vi "Create Array of Points.vi"(0 "rx output divider":T1, 5 "horizontal step size":i16=1, 7 "vertical step size":i16=1, 11 "error in":errorcluster) -> (4 "array of points":T2[][](array[typedef]), 15 "error out":errorcluster)   [LabVIEW 2014, in "niHighSpeedSerial Rectangular Eye Scan Point Iterator v1 Host.lvclass"]
doc: "Creates the array of points to measure based on the passed in parameters.\n\n<B>Input Parameters</B>\n\n<B>rx output divider</B> represents the configuration of the receiver output divider. This should match the values configured with RXRATE and RXOUT_DIV.\nenum values: 1,2,4,8,16\n\n<B>horizontal step size</B> is the number of offsets to skip between each point on the horizontal axis.\n\n<B>vertical step size</B> is the number of offsets to skip between each point on the vertical axis.\n\n<B>error in</B> describes error conditions that occur before this node runs. This input provides standard 'error in' functionality.\n\n<B>Output Parameters</B>\n\n<B>array of points</B> contains information related to each point, including its offsets, bit error rate, sample count, and error rate.\n\n<B>array of points.point offsets</B> contains the horizontal and vertical offsets for a point.\n\n<B>array of points.point offsets.horizontal offset</B> is the horizontal (unit interval) offset of a point.\n\n<B>array of points.point offsets.vertical offset</B> is the vertical (uncalibrated voltage) offset of a point.\n\n<B>array of points.sample count</B> is the number of samples measured.\n\n<B>array of points.error count</B> is the number of errors detected while measuring the point.\n\n<B>array of points.bit error rate</B> is the calculated statistical bit error rate based on the number of error counts and sample counts received.\n\n<B>error out</B> contains error information. This output provides standard 'error out' functionality."
uses:
  <instrlib>/niHighSpeedSerial/Eye Scan/v1/Host/Impl/Rect Iter/niHighSpeedSerial Rectangular Eye Scan Point Iterator v1 Host.lvclass
  <instrlib>/niHighSpeedSerial/Eye Scan/v1/Host/Common/Public/Point.ctl
  <instrlib>/niHighSpeedSerial/Eye Scan/v1/Host/Common/Public/Point Offsets.ctl
  <instrlib>/niHighSpeedSerial/Eye Scan/v1/Host/Common/Public/RX Output Divider.ctl
  <instrlib>/niHighSpeedSerial/Eye Scan/v1/Host/Common/niHighSpeedSerial Eye Scan Common v1 Host.lvlib
panel:
  out "size(s)":i32[](array[numeric])
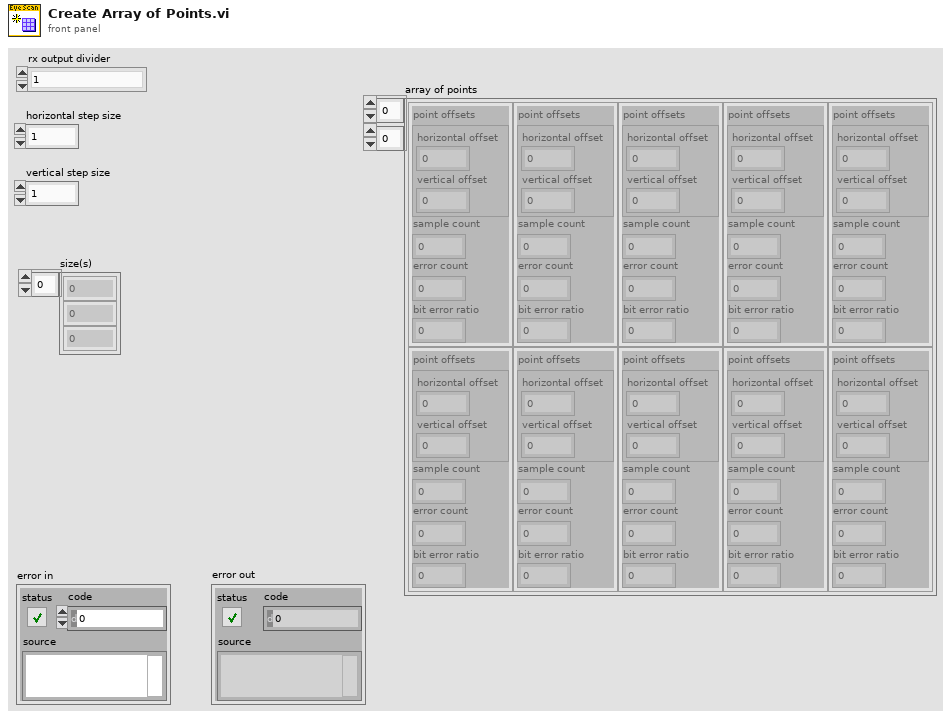
[diagram p1: front panel]
types:
  T1 = typedef "niHighSpeedSerial Eye Scan Common v1 Host.lvlib/RX Output Divider.ctl" = enum16{"1", "2", "4", "8", "16"}
  T2 = typedef "niHighSpeedSerial Eye Scan Common v1 Host.lvlib/Point.ctl" = cluster{"point offsets":T3, "sample count":u64, "error count":u64, "bit error ratio":dbl}
  T3 = typedef "niHighSpeedSerial Eye Scan Common v1 Host.lvlib/Point Offsets.ctl" = cluster{"horizontal offset":i16, "vertical offset":i8}
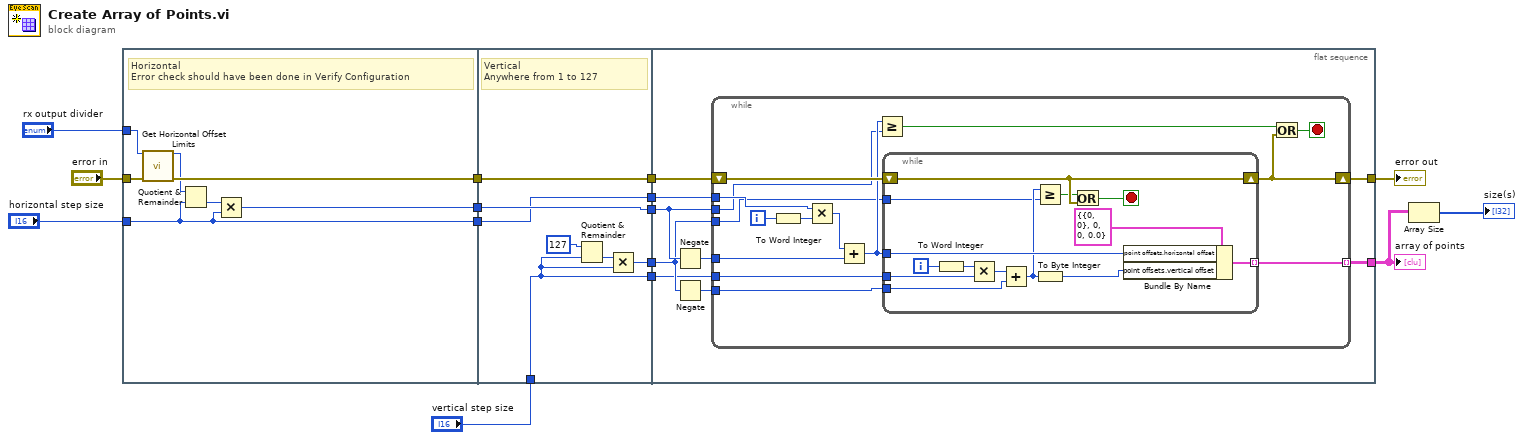
[diagram p0: block diagram]
diagram:
  n1 = flat-sequence {
    tunnel: "horizontal step size" -> [w17]
    tunnel: "rx output divider" -> [w19]
    tunnel: "error in" -> [w22]
    tunnel: [w17] -> w15
    tunnel: [w18] -> w8
    tunnel: [w21] -> w7
    tunnel: "vertical step size" -> [w23]
    tunnel: [w24] -> w14
    tunnel: w15 -> [w28]
    tunnel: w8 -> [w24]
    tunnel: w7 -> [w29]
    tunnel: [w29] -> w6
    tunnel: [w28] -> w3
    tunnel: [w26] -> w2
    tunnel: [w23] -> w1
    tunnel: [w35] -> w13
    tunnel: w14 -> [w36]
    tunnel: [w38] -> w4
    tunnel: w6 -> [w33]
    tunnel: w3 -> [w34]
    tunnel: w2 -> [w32]
    tunnel: w1 -> [w30]
    frame #0 {
      # "Horizontal\nError check should have been done in Verify Configuration"
      n2 = call <instrlib>:"Get Horizontal Offset Limits.vi"("rx output divider"=w19, "error in"=w22) -> ("maximum"=w16:i16, "error out"=w18:errorcluster)  [unwired: 10 in, 2 out]
      n3 = Quotient & Remainder(x=w16, y=w17) -> (floor(x/y)=w20:i16)  [unwired: 1 out]
      n4 = Multiply(x=w20, y=w17) -> (x*y=w21:i16)
    }
    frame #1 {
      # "Vertical\nAnywhere from 1 to 127"
      n5 = Quotient & Remainder(x=i16 127, y=w23) -> (floor(x/y)=w27:i16)  [unwired: 1 out]
      n6 = Multiply(x=w27, y=w23) -> (x*y=w26:i16)
    }
    frame #2 {
      n7 = Negate(x=w33) -> (-x=w37:i16)
      n8 = Negate(x=w32) -> (-x=w31:i16)
      n9 = while {
        tunnel: [w53] -> w38 mode=indexing
        tunnel: w37 -> [w46]
        shift-right: [w50] -> w35
        shift-left: w36 -> [w51]
        tunnel: w34 -> [w49]
        tunnel: w33 -> [w43]
        tunnel: w32 -> [w41]
        tunnel: w31 -> [w40]
        tunnel: w30 -> [w39]
        i -> [w48]
        stop <- w52 stop-if-true
        n10 = To Word Integer(number=w48) -> (16bit integer=w45:i16)
        n11 = Multiply(x=w49, y=w45) -> (x*y=w47:i16)
        n12 = Add(x=w47, y=w46) -> (x+y=w44:i16)
        n13 = Greater Or Equal?(x=w44, y=w43) -> (x >= y?=w42:bool)
        n14 = while {
          tunnel: [w67] -> w53 mode=indexing
          shift-right: [w65] -> w50
          shift-left: w51 -> [w65]
          tunnel: w44 -> [w64]
          tunnel: w41 -> [w57]
          tunnel: w40 -> [w59]
          tunnel: w39 -> [w61]
          i -> [w63]
          stop <- w66 stop-if-true
          n15 = To Word Integer(number=w63) -> (16bit integer=w62:i16)
          n16 = Multiply(x=w62, y=w61) -> (x*y=w60:i16)
          n17 = Add(x=w60, y=w59) -> (x+y=w58:i16)
          n18 = Greater Or Equal?(x=w58, y=w57) -> (x >= y?=w56:bool)
          n19 = To Byte Integer(number=w58) -> (8bit integer=w55:i8)
          n20 = Or(x=w56, y=w65) -> (x .or. y?=w66:bool)
          n21 = Bundle By Name(cluster=T2 {"point offsets"={"horizontal offset"=0, "vertical offset"=0}, "sample count"=0, "error count"=0, "bit error ratio"=0.0} ("point"), "point offsets.horizontal offset"=w64, "point offsets.vertical offset"=w55) -> (w67:T2)
        }
        n22 = Or(x=w42, y=w50) -> (x .or. y?=w52:bool)
      }
    }
  }
  n23 = Array Size(array=w4) -> (size(s)=→"size(s)":i32[])
  "array of points" <- w4
  "error out" <- w13
